vi "Assign Value.vi"(8 "error in (no error)":errorcluster, 10 "Assigned Value":refnum<class "Abs_Value.lvclass">, 11 "Abs_Double Float in":refnum<class "Abs_I32 Integer 1D.lvclass">) -> (0 "error out":errorcluster, 3 "Abs_Double Float out":refnum<class "Abs_I32 Integer 1D.lvclass">)   [LabVIEW 2021, in "Abs_I32 Integer 1D.lvclass"]
uses:
  Abs_I32 Integer 1D.lvclass
  Value/Abs_Value.lvclass
  Numeric 1D/Abs_Numeric_1D.lvclass
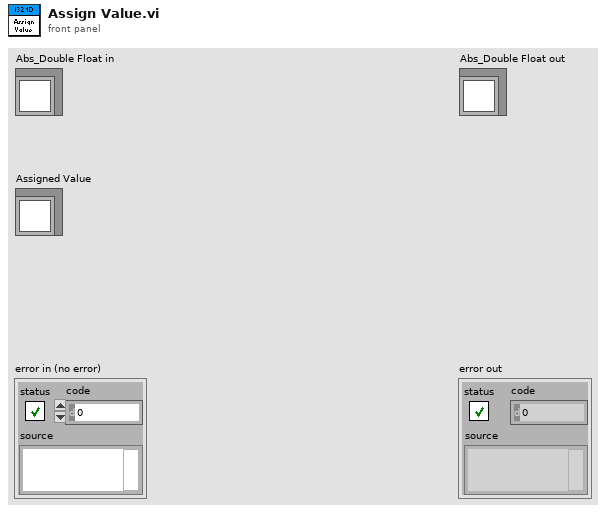
[diagram p1: front panel]
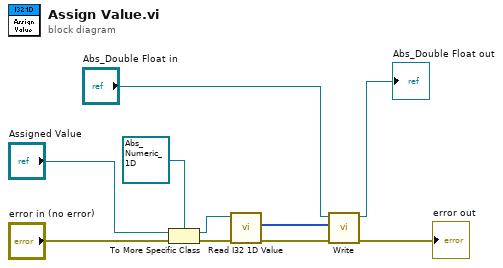
[diagram p0: block diagram]
diagram:
  n1 = To More Specific Class(target class=refnum<class "Abs_Numeric_1D.lvclass"> refnum ("Abs_Numeric_1D.lvclass"), reference="Assigned Value", error in="error in (no error)") -> (specific class reference=w2:refnum<class "Abs_Numeric_1D.lvclass">, error out=w4:errorcluster)
  n2 = call-dynamic "Read I32 1D Value.vi"("error in (no error)"=w4, "Numeric in"=w2) -> ("error out"=w3:errorcluster, "I32"=w1:i32[])  [unwired: 7 in, 1 out]
  n3 = call-dynamic "Write.vi"("error in (no error)"=w3, "Value"=w1, "Double Float.lvclass in"="Abs_Double Float in") -> ("error out"=→"error out":errorcluster, "Double Float.lvclass out"=→"Abs_Double Float out":refnum<class "Abs_I32 Integer 1D.lvclass">)  [unwired: 7 in]
